vi "Write Inherit Tests_.vi"(8 "error in (no error)":errorcluster, 10 "Inherit Tests?":bool, 11 "Process Generator In":refnum<class "Process Generator.lvclass">) -> (0 "error out":errorcluster, 3 "Process Generator Out":refnum<class "Process Generator.lvclass">)   [LabVIEW 2020, in "Process Generation.lvlib" / "Process Generator.lvclass"]
uses:
  Process Generator.lvclass
  Process Generator.lvclass/Process Generator.ctl
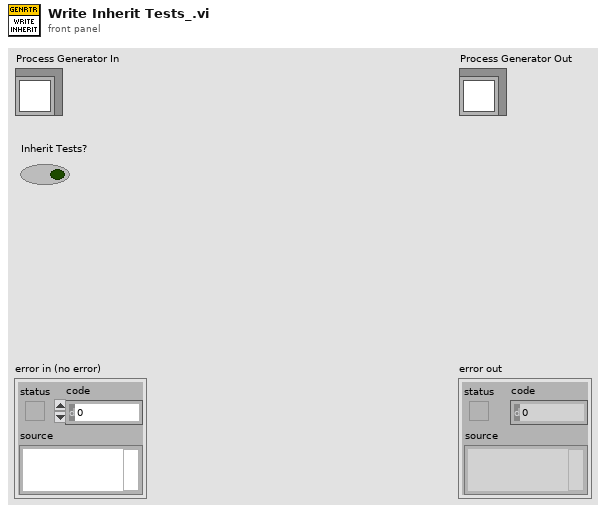
[diagram p1: front panel]
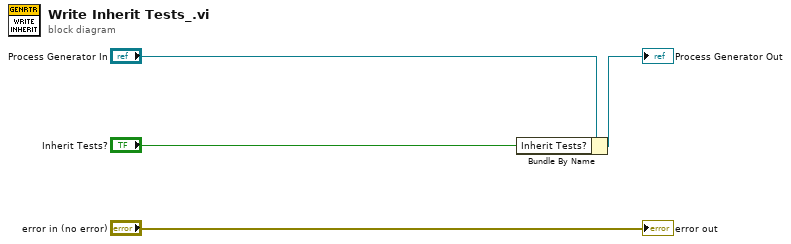
[diagram p0: block diagram]
diagram:
  n1 = Bundle By Name(cluster="Process Generator In", "Inherit Tests?"="Inherit Tests?") -> (→"Process Generator Out":refnum<class "Process Generator.lvclass">)
  "error out" <- "error in (no error)"
